vi "Side distances.vi"(5 "Heading":dbl, 6 "side back":dbl, 7 "side front":dbl) -> (0 "side front y":i32, 1 "side back x":i32, 2 "side front y":i32, 3 "side front x":i32)   [LabVIEW 2015]
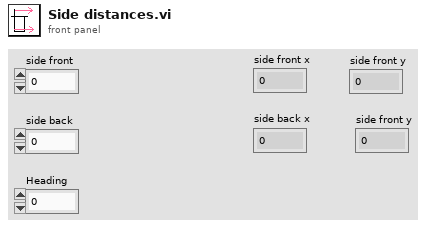
[diagram p1: front panel]
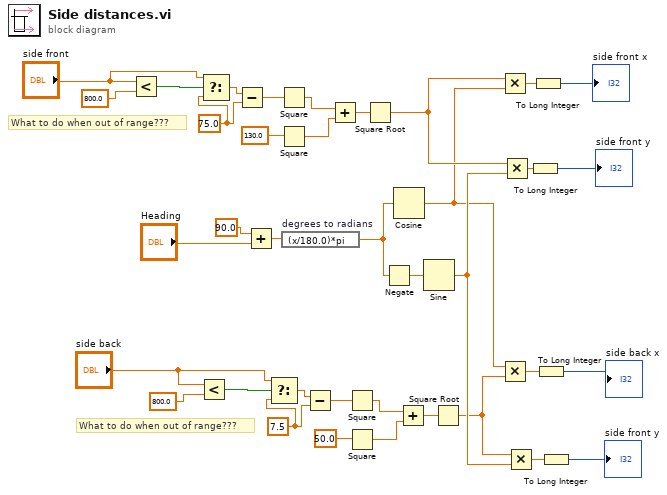
[diagram p0: block diagram]
diagram:
  w14 = 7.5 ("y")
  w26 = 75.0 ("y")
  # "What to do when out of range???"
  # "What to do when out of range???"
  n1 = Less?(x="side front", y=800.0) -> (x < y?=w29:bool)
  n2 = Less?(x="side back", y=800.0) -> (x < y?=w16:bool)
  n3 = Select(t="side front", s=w29, f=w26) -> (s? t:f=w25:dbl)
  n4 = Subtract(x=w25, y=w26) -> (x-y=w33:dbl)
  n5 = Add(x=90.0, y="Heading") -> (x+y=w36:dbl)
  n6 = Select(t="side back", s=w16, f=w14) -> (s? t:f=w13:dbl)
  n7 = Square(x=w33) -> (x^2=w31:dbl)
  n8 = Square(x=130.0) -> (x^2=w30:dbl)
  n9 = expression code="(x/180.0)*pi" "degrees to radians"(w36) -> (w37:dbl)
  n10 = Subtract(x=w13, y=w14) -> (x-y=w20:dbl)
  n11 = Add(x=w31, y=w30) -> (x+y=w24:dbl)
  n12 = Square(x=w20) -> (x^2=w18:dbl)
  n13 = Square(x=50.0) -> (x^2=w17:dbl)
  n14 = Square Root(x=w24) -> (sqrt(x)=w21:dbl)
  n15 = Negate(x=w37) -> (-x=w1:dbl)
  n16 = Cosine(x=w37) -> (cos(x)=w7:dbl)
  n17 = Add(x=w18, y=w17) -> (x+y=w12:dbl)
  n18 = Sine(x=w1) -> (sin(x)=w8:dbl)
  n19 = Square Root(x=w12) -> (sqrt(x)=w6:dbl)
  n20 = Multiply(x=w21, y=w7) -> (x*y=w23:dbl)
  n21 = Multiply(x=w7, y=w6) -> (x*y=w10:dbl)
  n22 = Multiply(x=w21, y=w8) -> (x*y=w22:dbl)
  n23 = Multiply(x=w6, y=w8) -> (x*y=w9:dbl)
  n24 = To Long Integer(number=w22) -> (32bit integer=→"side front y":i32)
  n25 = To Long Integer(number=w23) -> (32bit integer=→"side front x":i32)
  n26 = To Long Integer(number=w10) -> (32bit integer=→"side back x":i32)
  n27 = To Long Integer(number=w9) -> (32bit integer=→"side front y":i32)
